vi "CfgClkRef.vi"(8 "error in (no error)":errorcluster, 11 "NiPxi6683H":refnum<class "NiPxi6683H.lvclass">) -> (0 "error out":errorcluster, 3 "NiPxi6683H":refnum<class "NiPxi6683H.lvclass">)   [LabVIEW 2014, in "SyncPlugins.lvlib" / "NiPxi6683H.lvclass"]
uses:
  NiPxi6683H.lvclass
  NiPxi6683H.lvclass/NiPxi6683H.ctl
  NiPxi6682/NiPxi6682.lvclass/NiPxi6682.ctl
  SyncPluginBase/SyncPluginBase.lvclass/SyncPluginBase.ctl
  Accessors/Read TimeRefType.vi
  NiPxi6682/Accessors/Write NiSyncHandle.vi
  SyncPluginBase/Accessors/Write Initiated.vi
  SyncPluginBase/Accessors/Write Locked.vi
  SyncPluginBase/Accessors/Write Run.vi
  NiPxi6682/Accessors/Write SysHandle.vi
  NiPxi6682/Accessors/Write SysRef.vi
  NiPxi6682/Accessors/Read NiSyncHandle.vi
  <instrlib>/niSync/niSync.llb/niSync Initialize (IVI).vi
  <instrlib>/niSync/niSync.llb/niSync Set Time Reference (GPS).vi
  <instrlib>/niSync/niSync.llb/niSync Set Time Reference (IRIG).vi
  <instrlib>/niSync/niSync.llb/niSync Set Time Reference (Free Running).vi
  <instrlib>/niSync/niSync.llb/niSync Set Time Reference (1588 Ordinary Clock).vi
  <instrlib>/niSync/niSync.llb/niSync Set Time Reference (PPS).vi
  <vilib>/nisyscfg/nisyscfg.lvlib
  <resource>/objmgr/niMIDebugSession.rc
  <resource>/objmgr/nisysapi.rc
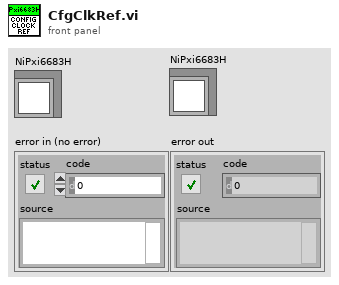
[diagram p1: front panel]
types:
  T1 = typedef "SyncPlugins.lvlib/PXI_MultiTrig.lvclass/TimeRefType.ctl" = enum16{"1588", "Free Running", "GPS", "IRIG", "PPS"}
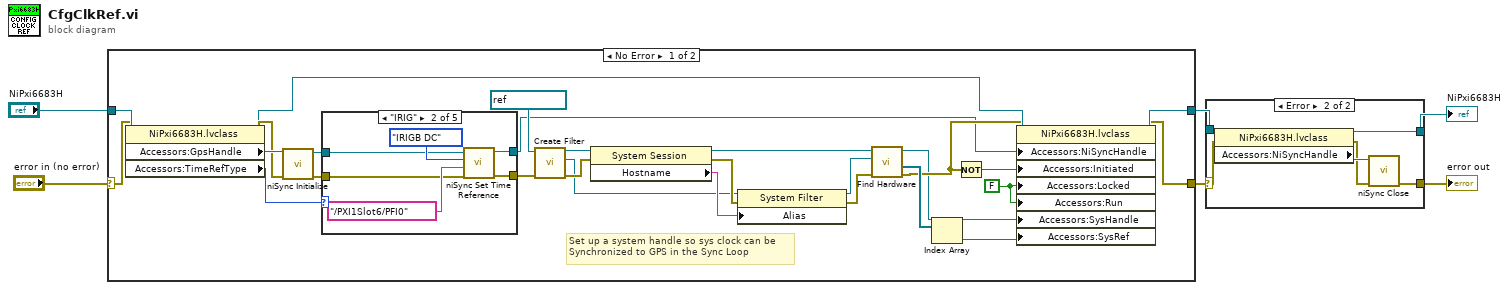
[diagram p0: block diagram]
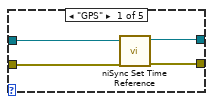
[diagram p3: hidden frame]
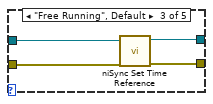
[diagram p4: hidden frame]
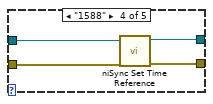
[diagram p5: hidden frame]
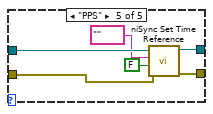
[diagram p6: hidden frame]
diagram:
  n1 = case shown="No Error" "error in (no error)" {
    selector: "error in (no error)" -> [w32 w58]
    tunnel: "NiPxi6683H" -> [w33 w59]
    tunnel: [w10 w59] -> w4
    tunnel: [w9 w58] -> w2
    frame No Error {
      w13 = FALSE
      # "Set up a system handle so sys clock can be\nSynchronized to GPS in the Sync Loop"
      n2 = property class="NiPxi6683H.lvclass"(reference=w33, error in=w32) -> (reference out=w16:refnum<class "NiPxi6683H.lvclass">, error out=w30:errorcluster, "Accessors:GpsHandle"=w31:refnum<k15>, "Accessors:TimeRefType"=w8:T1)
      n3 = call-poly <instrlib>:"niSync Initialize.vi"("error in (no error)"=w30, "resource name"=w31) -> ("error out"=w29:errorcluster, "instrument handle out"=w28:refnum<k15>)  [unwired: 8 in]
      n4 = case shown="\"IRIG\"" w8 {
        tunnel: w29 -> [w37 w38 w47 w51 w52]
        tunnel: w28 -> [w36 w39 w46 w50 w55]
        tunnel: [w35 w43 w45 w49 w57] -> w18
        tunnel: [w34 w42 w44 w48 w56] -> w7
        frame "GPS" {
          n5 = call-poly <instrlib>:"niSync Set Time Reference.vi"("error in (no error)"=w37, "instrument handle"=w36) -> ("error out"=w35:errorcluster, "instrument handle out"=w34:refnum<k15>)  [unwired: 8 in]
        }
        frame "IRIG" {
          n6 = call-poly <instrlib>:"niSync Set Time Reference.vi"("error in (no error)"=w38, "terminal"=tag "/PXI1Slot6/PFI0", "IRIG type"=enum16{"IRIGB DC", "IRIGB AM"}."IRIGB DC", "instrument handle"=w39) -> ("error out"=w43:errorcluster, "instrument handle out"=w42:refnum<k15>)  [unwired: 6 in]
        }
        frame "Free Running", Default {
          n7 = call-poly <instrlib>:"niSync Set Time Reference.vi"("error in (no error)"=w47, "instrument handle"=w46) -> ("error out"=w45:errorcluster, "instrument handle out"=w44:refnum<k15>)  [unwired: 8 in]
        }
        frame "1588" {
          n8 = call-poly <instrlib>:"niSync Set Time Reference.vi"("error in (no error)"=w51, "instrument handle"=w50) -> ("error out"=w49:errorcluster, "instrument handle out"=w48:refnum<k15>)  [unwired: 8 in]
        }
        frame "PPS" {
          n9 = call-poly <instrlib>:"niSync Set Time Reference.vi"("error in (no error)"=w52, "use manual time"=FALSE, "terminal"=tag "", "instrument handle"=w55) -> ("error out"=w57:errorcluster, "instrument handle out"=w56:refnum<k15>)  [unwired: 6 in]
        }
      }
      n10 = call <vilib>:"Create Filter.vi"("error in (no error)"=w18, "Session in"=refnum<k21> "localhost") -> ("error out"=w26:errorcluster, "Filter out"=w19:refnum<k20>, "Session out"=w20:refnum<k21>)  [unwired: 7 in]
      n11 = property class="System Session"(reference=w20, error in=w26) -> (reference out=w22:refnum<k21>, error out=w27:errorcluster, "Hostname"=w21:string)
      n12 = property class="System Filter"(reference=w19, error in=w27, "Alias"=w21) -> (reference out=w23:refnum<k20>, error out=w24:errorcluster)
      n13 = call <vilib>:"Find Hardware.vi"("error in (no error)"=w24, "Filter in"=w23, "Session in"=w22) -> ("error out"=w15:errorcluster, "Resources out"=w25:refnum<k20>[], "Session out"=w11:refnum<k21>)  [unwired: 5 in, 1 out]
      n14 = Index Array(array=w25) -> (element=w12:refnum<k20>)  [unwired: 1 in]
      n15 = Not(x=w15) -> (.not. x?=w14:bool)
      n16 = property class="NiPxi6683H.lvclass"(reference=w16, error in=w15, "Accessors:NiSyncHandle"=w7, "Accessors:Initiated"=w14, "Accessors:Locked"=w13, "Accessors:Run"=w13, "Accessors:SysHandle"=w11, "Accessors:SysRef"=w12) -> (reference out=w10:refnum<class "NiPxi6683H.lvclass">, error out=w9:errorcluster)
    }
    frame Error {
    }
  }
  n17 = case shown="Error" w2 {
    selector: w2 -> [w60 w64]
    tunnel: w4 -> [w61 w67]
    tunnel: [w61 w66] -> w3
    tunnel: [w60 w62] -> w1
    frame No Error {
    }
    frame Error {
      n18 = property class="NiPxi6683H.lvclass"(reference=w67, error in=w64) -> (reference out=w66:refnum<class "NiPxi6683H.lvclass">, error out=w63:errorcluster, "Accessors:NiSyncHandle"=w65:refnum<k15>)
      n19 = call <instrlib>:"niSync Close.vi"("error in (no error)"=w63, "instrument handle"=w65) -> ("error out"=w62:errorcluster)  [unwired: 9 in]
    }
  }
  "NiPxi6683H" <- w3
  "error out" <- w1
